vi "E3L_IDC.vi"(11 "IDC in":i32) -> (3 "IDC out":dbl)   [LabVIEW 2022 SP3]
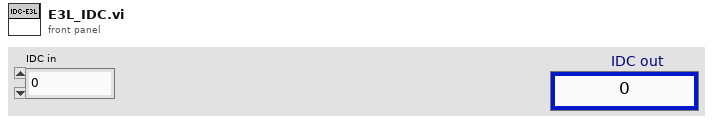
[diagram p1: front panel]
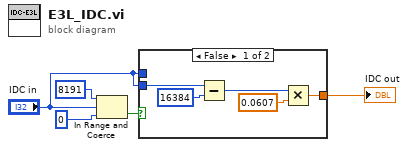
[diagram p0: block diagram]
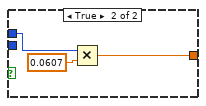
[diagram p2: hidden frame]
diagram:
  n1 = In Range and Coerce(upper limit=8191, x="IDC in", lower limit=0) -> (In Range?=w3:bool)  [unwired: 1 out]
  n2 = case shown="False" w3 {
    tunnel: "IDC in" -> [w10 _]
    tunnel: "IDC in" -> [_ w11]
    tunnel: [w6 w12] -> w1
    frame False {
      n3 = Subtract(x=w10, y=16384) -> (x-y=w8:i32)
      n4 = Multiply(x=w8, y=0.0607) -> (x*y=w6:dbl)
    }
    frame True {
      n5 = Multiply(x=w11, y=0.0607) -> (x*y=w12:dbl)
    }
  }
  "IDC out" <- w1
